vi "PrepareDataForParserSorter.vi"(8 "Error In":errorcluster, 11 "SRList":T6 {"SR#" format="%#_10g"}) -> (0 "Error Out":errorcluster, 3 "Prepared SR List":T1[](array[typedef]))   [LabVIEW 2017, in "Client.lvlib"]
uses:
  Client.lvlib
  ServerCommunications/TypeDefs/SRList.ctl
  ServerCommunications/TypeDefs/SRData.ctl
  ParserSorter/TypeDefs/SRData.ctl
  ParserSorter/TypeDefs/AEGroup.ctl
  ParserSorter/TypeDefs/SRStatus.ctl
  ParserSorter/TypeDefs/SRLevel.ctl
  ParserSorter/TypeDefs/SRType.ctl
  ParserSorter/ParserSorter.lvlib
  ServerCommunications/CommsServer.lvlib
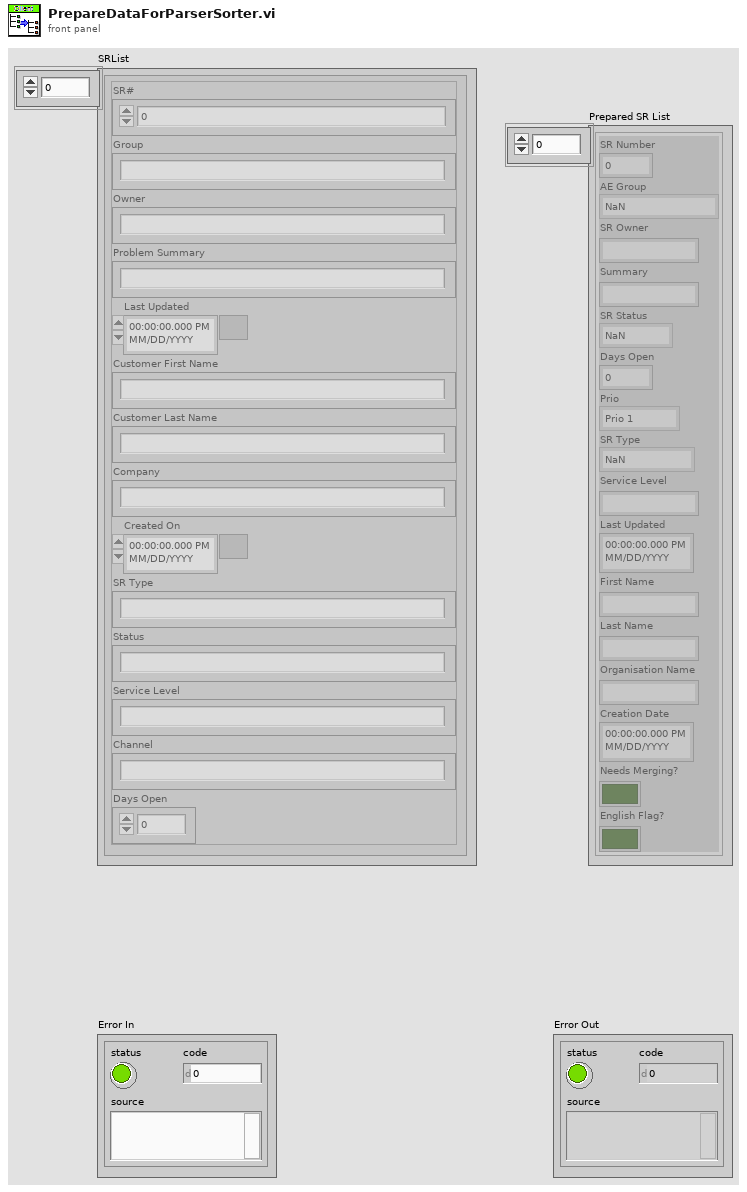
[diagram p1: front panel]
types:
  T1 = typedef "Client.lvlib/ParserSorter.lvlib/SRData.ctl" = cluster{"SR Number":i64, "AE Group":T2, "SR Owner":string, "Summary":string, "SR Status":T3, "Days Open":dbl, "Prio":T4, "SR Type":T5, "Service Level":string, "Last Updated":timestamp, "First Name":string, "Last Name":string, "Organisation Name":string, "Creation Date":timestamp, "Needs Merging?":bool, "English Flag?":bool}
  T2 = typedef "Client.lvlib/ParserSorter.lvlib/AEGroup.ctl" = enum32{"NaN", "AE-Germany", "AE-Poland", "AE-Switzerland", "AE-Czech Republic", "AE-Hungary", "AE-Romania", "AE-Slovakia", "AE-Slovenia"}
  T3 = typedef "Client.lvlib/ParserSorter.lvlib/SRStatus.ctl" = enum32{"NaN", "Caller Abandoned", "Created in Error", "Declined to Purchase Support", "Expired", "Forum Resolved AE", "Forum Resolved Customer", "IN WORK", "IN WORK Collab with AES", "IN WORK Collab with PSE", "IN WORK Collab with SE", "IN WORK Escalation", "IN WORK Customer Added Note", "Open", "Potentially Resolved", "POC Resolved", "Resolved", "RMA Waiting on Customer", "RMA Open", "RMA In Progress", "RMA Closed - DOA", "RMA Closed", "RMA Approved for Return", "Project Complete", "Presumed Resolved", "IN WORK Wait on Customer"}
  T4 = typedef "Client.lvlib/ParserSorter.lvlib/SRLevel.ctl" = enum16{"Prio 1", "Prio 2", "Prio 3", "Prio 4"}
  T5 = typedef "Client.lvlib/ParserSorter.lvlib/SRType.ctl" = enum32{"NaN", "ATE Core Configurations (BYOATE)", "Activation", "BioBench", "CAN", "CM C Series", "Calibration", "Consulting Services", "CounterTimer", "DAQExpress", "DASYLab", "DIAdem", "DMM", "DSA HW", "Digital_IO", "FIRST (NIC Only)", "FieldBus", "FieldPoint", "Functional Savety", "GATI", "GPIB", "HMI and Industrial PCs", "HiQ", "HighSpeedDigital_IO", "IMAQ", "IOTech Vibration", "Industrial Communications", "InsightCM", "LV", "LV CD&Sim", "LV Comms", "LV Controls Add-Ons", "LV Embedded", "LV MathScript RT", "LV NXG", "LV NXT", "LVDSC", "LVFPGA", "LVPDA and LV Touch Panel", "LVRT", "LabWindows_CVI", "Lookout", "MATRIXx", "MStudioDotNet", "MStudioVisualBasic", "MStudioVisualC", "Measure (Legacy)", "Motion", "MultifunctionDAQ", "Multimedia Test HW/SW", "Multisim (EWB)", "NI Update Service", "OPC Servers", "Optical (OSI)", "PXI Controllers, Chassis, MXI", "PXI Timing and Sync", "Power Supplies and SMUs", "Powertrain Controls", "RAID", "RF", "RF Software", "RIO", "SC Express", "SCC", "SCXI", "SPEEDY-33 (Hyperception)", "STS", "ScopeDigitizers", "Serial", "Signal Sources", "SignalCondOther", "SignalExpress", "Software Defined Intruments", "Sound and Vibration SW", "Switch Executive", "Switches", "TestStand", "USRP", "Ultiboard (EWB)", "VBench", "VI Logger", "VXI_MXI", "VeriStand", "VisionSW", "VolumeLicenseMgr", "WSN", "Web UI Builder", "myRIO"}
  T6 = typedef "Client.lvlib/CommsServer.lvlib/SRList.ctl" = T7[]
  T7 = typedef "Client.lvlib/CommsServer.lvlib/SRData.ctl" = cluster{"SR#":dbl, "Group":string, "Owner":string, "Problem Summary":string, "Last Updated":timestamp, "Customer First Name":string, "Customer Last Name":string, "Company":string, "Created On":timestamp, "SR Type":string, "Status":string, "Service Level":string, "Channel":string, "Days Open":dbl}
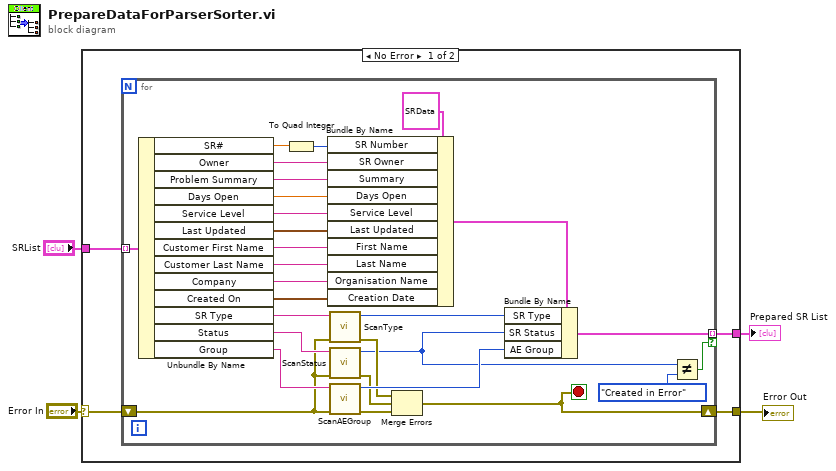
[diagram p0: block diagram]
diagram:
  n1 = case shown="No Error" "Error In" {
    selector: "Error In" -> [w6 w37]
    tunnel: [w5 w37] -> w3
    tunnel: "SRList" -> [w8 _]
    tunnel: [w7 _] -> w1
    frame No Error {
      n2 = for {
        tunnel: w8 -> [w36] mode=indexing
        tunnel: [w21] -> w7 mode=indexing if=w11
        shift-right: [w14] -> w5
        shift-left: w6 -> [w16]
        stop <- w14 stop-if-true
        n3 = Unbundle By Name(w36) -> ("SR#"=w33:dbl, "Owner"=w31:string, "Problem Summary"=w30:string, "Days Open"=w29:dbl, "Service Level"=w28:string, "Last Updated"=w27:timestamp, "Customer First Name"=w26:string, "Customer Last Name"=w25:string, "Company"=w24:string, "Created On"=w23:timestamp, "SR Type"=w18:string, "Status"=w22:string, "Group"=w20:string)
        n4 = To Quad Integer(1:w33) -> (0:w32:i64)
        n5 = Bundle By Name(cluster=T1 {"SR Number"=0, "AE Group"=enum."NaN", "SR Owner"="", "Summary"="", "SR Status"=enum."Open", "Days Open"=0.0, "Prio"=enum."Prio 1", "SR Type"=enum."OPC Servers", "Service Level"="", "Last Updated"=timestamp(0 s since 1904-01-01), "First Name"="", "Last Name"="", "Organisation Name"="", "Creation Date"=timestamp(0 s since 1904-01-01), "Needs Merging?"=FALSE, "English Flag?"=FALSE} ("SR Number"), "SR Number"=w32, "SR Owner"=w31, "Summary"=w30, "Days Open"=w29, "Service Level"=w28, "Last Updated"=w27, "First Name"=w26, "Last Name"=w25, "Organisation Name"=w24, "Creation Date"=w23) -> (w34:T1)
        n6 = call "ScanType.vi"("error in (no error)"=w16, "Type String"=w18) -> ("error out"=w12:errorcluster, "SR Type"=w17:T5)  [unwired: 8 in]
        n7 = call "ScanStatus.vi"("error in (no error)"=w16, "Status String"=w22) -> ("error out"=w13:errorcluster, "SR Status"=w10:T3)  [unwired: 8 in]
        n8 = call "ScanAEGroup.vi"("error in (no error)"=w16, "AE Group String"=w20) -> ("error out"=w15:errorcluster, "AE Group"=w19:T2)  [unwired: 8 in]
        n9 = Merge Errors(w12, w13, w15) -> (w14:errorcluster)
        n10 = Bundle By Name(cluster=w34, "SR Type"=w17, "SR Status"=w10, "AE Group"=w19) -> (w21:T1)
        n11 = Not Equal?(x=w10, y=SRStatus."Created in Error") -> (x != y?=w11:bool)
      }
    }
    frame Error {
    }
  }
  "Error Out" <- w3
  "Prepared SR List" <- w1
